vi "File_Read Write Icon Template colors.vi"(6 "Read(f)\nWrite(t)":bool, 8 "Error":errorcluster, 9 "Home Path":path, 11 "Template Select":T1[](array[typedef]) {"Format"."Icon Sizing"."Rows" min=1 max=5 step=1; "Format"."Icon Sizing"."Width" min=7 max=32 step=1}) -> (0 "Error Out":errorcluster, 2 "Final Path Out":path, 3 "Template Select Out":T1[](array[typedef]) {"Format"."Icon Sizing"."Rows" min=1 max=5 step=1; "Format"."Icon Sizing"."Width" min=7 max=32 step=1})   [LabVIEW 2009]
doc: "Read or Write Icon template history file"
uses:
  Controls/Cluster/Cluster_Format Storage.ctl
  Controls/String_Picture/STRING_Line Display.ctl
  Controls/Cluster/Cluster_Icon Format.ctl
  Controls/Cluster/Cluster_Icon Color Set.ctl
  Controls/Enum/ENUM_Frame Template Select.ctl
  Controls/Cluster/Cluster_Sizing Data.ctl
  Controls/Enum/ENUM_Icon Sizing.ctl
  Controls/Enum/RBENUM_Icon Position.ctl
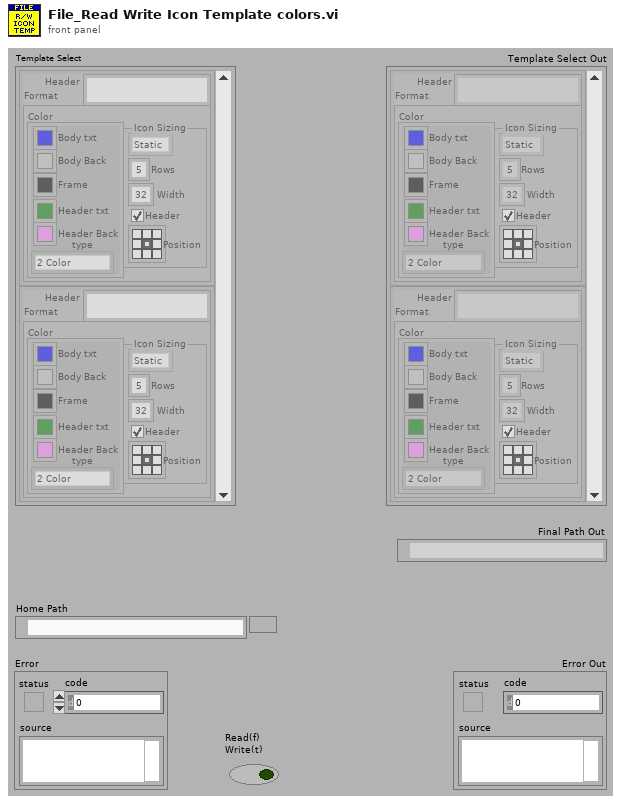
[diagram p1: front panel]
types:
  T1 = typedef "Cluster_Format Storage.ctl" = cluster{"Header":T2, "Format":T3}
  T2 = typedef "STRING_Line Display.ctl" = string
  T3 = typedef "Cluster_Icon Format.ctl" = cluster{"Color":T4, "Icon Sizing":T6}
  T4 = typedef "Cluster_Icon Color Set.ctl" = cluster{"Body txt":u32, "Body Back":u32, "Frame":u32, "Header txt":u32, "Header Back":u32, "type":T5}
  T5 = typedef "ENUM_Frame Template Select.ctl" = enum16{"2 Color", "5 Color"}
  T6 = typedef "Cluster_Sizing Data.ctl" = cluster{"Rule":T7, "Header":bool, "Rows":u32, "Width":u32, "Position":T8}
  T7 = typedef "ENUM_Icon Sizing.ctl" = enum16{"Static", "Auto"}
  T8 = typedef "RBENUM_Icon Position.ctl" = enum32{"LFT-TOP", "MID-TOP", "RGT-TOP", "LFT-CTR", "MID-CTR", "RGT-CTR", "LFT-BOT", "MID-BOT", "RGT-BOT"}
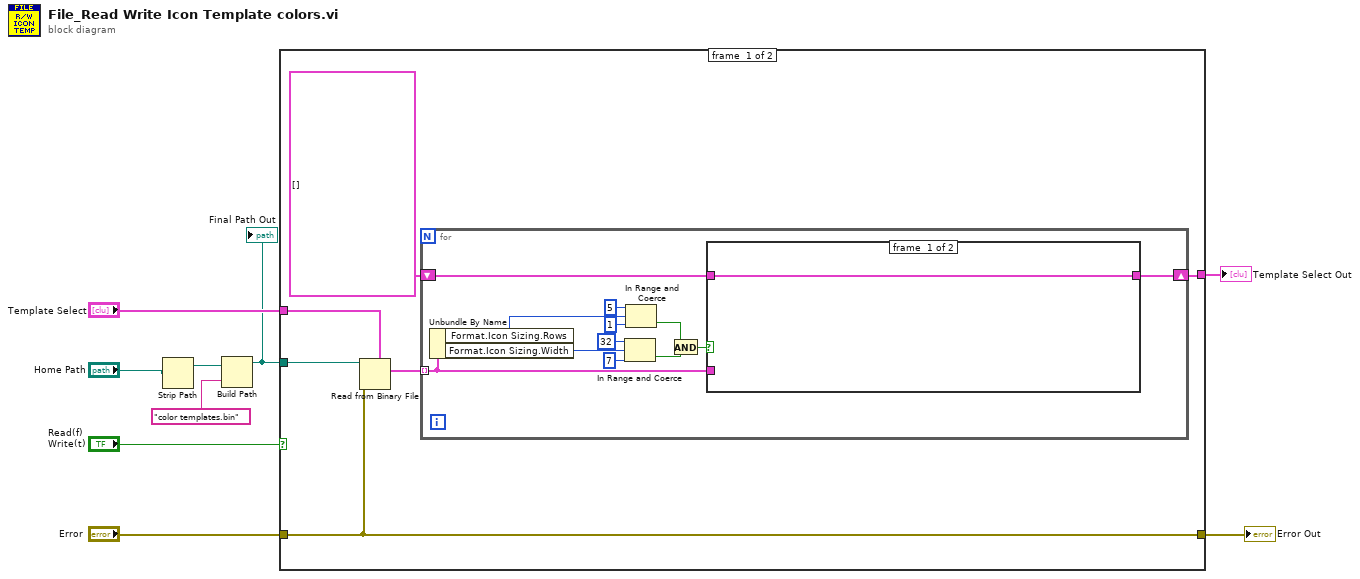
[diagram p0: block diagram]
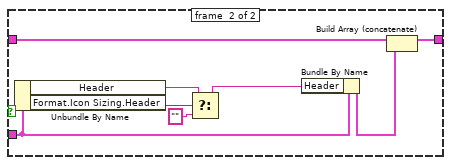
[diagram p2: hidden frame]
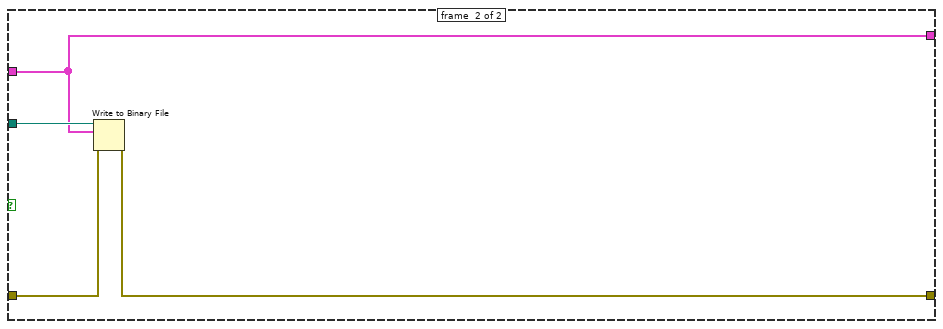
[diagram p3: hidden frame]
diagram:
  n1 = Strip Path(path="Home Path") -> (stripped path=w3:path)  [unwired: 1 out]
  n2 = Build Path(base path=w3, name or relative path="color templates.bin") -> (appended path=w5:path)
  "Final Path Out" <- w5
  n3 = case shown="False" "Read(f)\nWrite(t)" {
    tunnel: [w13 w40] -> w9
    tunnel: "Error" -> [w13 w39]
    tunnel: "Template Select" -> [w14 w37]
    tunnel: w5 -> [w15 w38]
    tunnel: [w11 w37] -> w1
    frame #0 {
      n4 = Read from Binary File(5:w14, 8:w13, 11:w15) -> (2:w12:T1[])  [unwired: 3 in, 3 out]
      n5 = for {
        tunnel: w12 -> [w27] mode=indexing
        shift-right: [w24] -> w11
        shift-left: T1[] [] -> [w25]
        n6 = Unbundle By Name(w27) -> ("Format.Icon Sizing.Rows"=w22:u32, "Format.Icon Sizing.Width"=w23:u32)
        n7 = In Range and Coerce(upper limit=u32 32, x=w23, lower limit=u32 7) -> (In Range?=w21:bool)  [unwired: 1 out]
        n8 = In Range and Coerce(upper limit=u32 5, x=w22, lower limit=u32 1) -> (In Range?=w20:bool)  [unwired: 1 out]
        n9 = And(x=w20, y=w21) -> (x .and. y?=w26:bool)
        n10 = case shown="True" w26 {
          tunnel: w27 -> [_ w31]
          tunnel: w25 -> [w28 w36]
          tunnel: [w28 w35] -> w24
          frame #0 {
          }
          frame #1 {
            n11 = Unbundle By Name(w31) -> ("Header"=w33:T2, "Format.Icon Sizing.Header"=w34:bool)
            n12 = Select(t=w33, s=w34, f=T2 "") -> (s? t:f=w29:T2)
            n13 = Bundle By Name(cluster=w31, "Header"=w29) -> (w30:T1)
            n14 = Build Array (concatenate)(w36, w30) -> (w35:T1[])
          }
        }
      }
    }
    frame #1 {
      n15 = Write to Binary File(file (use dialog)=w38, data=w37, error in=w39) -> (error out=w40:errorcluster)  [unwired: 3 in, 2 out]
    }
  }
  "Error Out" <- w9
  "Template Select Out" <- w1
